vi "RAW-Streamed Data to File per Channels.vi"(8 "error in (no error)":errorcluster) -> (0 "error out":errorcluster)   [LabVIEW 2016]
uses:
  Chennales to Process Custer.ctl
panel:
  in  "Start":bool
  in  "Chennales to Process":T1
  in  "Raw Data File Path":path
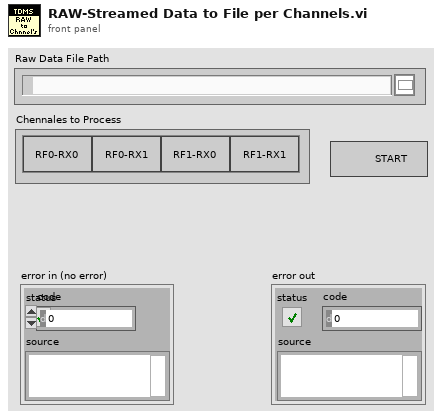
[diagram p1: front panel]
types:
  T1 = typedef "Chennales to Process Custer.ctl" = cluster{"RF0-RX0":bool, "RF0-RX1":bool, "RF1-RX0":bool, "RF1-RX1":bool}
  T2 = enum16{"open", "open or create", "create or replace", "create", "open (read-only)"}
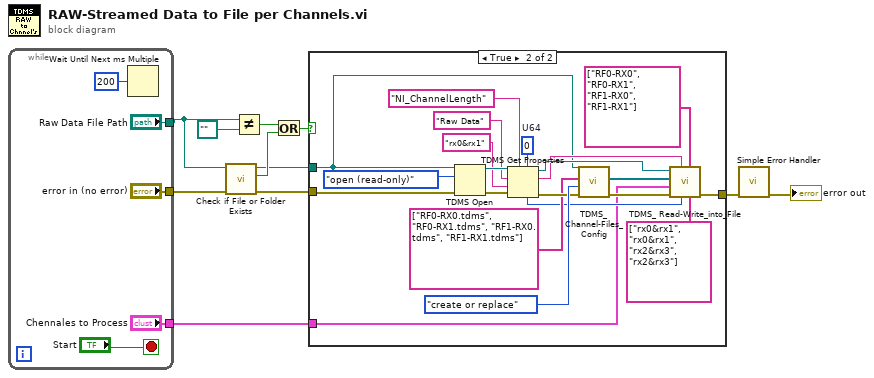
[diagram p0: block diagram]
diagram:
  n1 = while {
    tunnel: ["Raw Data File Path"] -> w3
    tunnel: ["Chennales to Process"] -> w2
    tunnel: ["error in (no error)"] -> w1
    stop <- "Start" stop-if-true
    n2 = Wait Until Next ms Multiple(millisecond multiple=u32 200) -> ()  [unwired: 1 out]
  }
  n3 = call <vilib>:"Check if File or Folder Exists.vi"("error in (no error)"=w1, "path"=w3) -> ("error out"=w8:errorcluster, "file or folder exists?"=w9:bool, "dup path"=w7:path)  [unwired: 7 in]
  n4 = Not Equal?(x=w3, y=path "") -> (x != y?=w10:bool)
  n5 = Or(x=w10, y=w9) -> (x .or. y?=w6:bool)
  n6 = case shown="True" w6 {
    tunnel: w8 -> [w17 w38]
    tunnel: w7 -> [_ w23]
    tunnel: [w17 w24] -> w5
    tunnel: w2 -> [_ w18]
    frame False {
    }
    frame True {
      w32 = u64 0  # U64
      n7 = TDMS Open(8:w38, 10:T2."open (read-only)" ("operation (0:open)"), 11:w23) -> (0:w34:errorcluster, 3:w35:refnum<k34>)  [unwired: 4 in]
      n8 = TDMS Get Properties(5:w32, 7:"NI_ChannelLength" ("Eigenschaftsname"), 8:w34, 9:"rx0&rx1" ("Kanalnamen (Eingang)"), 10:"Raw Data" ("Gruppenname (Eingang)"), 11:w35) -> (0:w30:errorcluster, 2:w26:string, 3:w31:refnum<k34>, 4:w20:u64)  [unwired: 2 out]
      n9 = call "TDMS_Channel-Files_Config.vi"("Error in"=w30, "File operation (0:open)"=T2."create or replace" ("operation (0:open)"), "File Names Array"=string[] ["RF0-RX0.tdms", "RF0-RX1.tdms", "RF1-RX0.tdms", "RF1-RX1.tdms"], "stripped path"=w23) -> ("Error out"=w29:errorcluster, "TDMS Write File Reference Array"=w21:refnum<k34>[])  [unwired: 6 in]
      n10 = call "TDMS_ Read-Write_into_File.vi"("Channel Names to Read"=string[] ["rx0&rx1", "rx0&rx1", "rx2&rx3", "rx2&rx3"], "Channel Names to Write"=string[] ["RF0-RX0", "RF0-RX1", "RF1-RX0", "RF1-RX1"], "Number of Values in Raw Channel"=w20, "group name"=w26, "Error in"=w29, "Chennales to Process"=w18, "TDMS Write Files References"=w21, "TDMS Raw-File Reference"=w31) -> ("Error out"=w24:errorcluster)  [unwired: 3 in]
    }
  }
  n11 = call <vilib>:"Simple Error Handler.vi"("error in (no error)"=w5) -> ("error out"=→"error out":errorcluster)  [unwired: 4 in, 4 out]
